vi "Lab4 prelab.vi"() -> ()   [LabVIEW 2016]
uses:
  <vilib>/Analysis/1siggen.llb/Ramp Pattern by Samples.vi
  <vilib>/Analysis/NI_AALBase.lvlib
panel:
  out "V":dbl
  out "I":dbl
  out "Data Length":dbl
  out "XY Graph":cluster{"Y":dbl[], "Y":dbl[]}[](graph)
  in  "V_D step [V]":dbl
  in  "V_D stop [V]":dbl
  in  "V_D start [V]":dbl
  in  "R":dbl
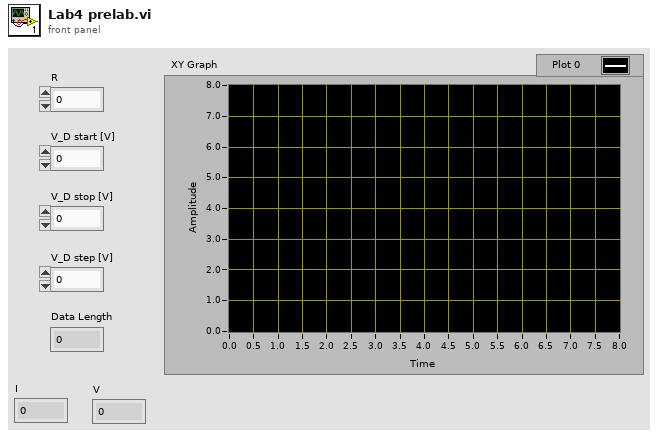
[diagram p1: front panel]
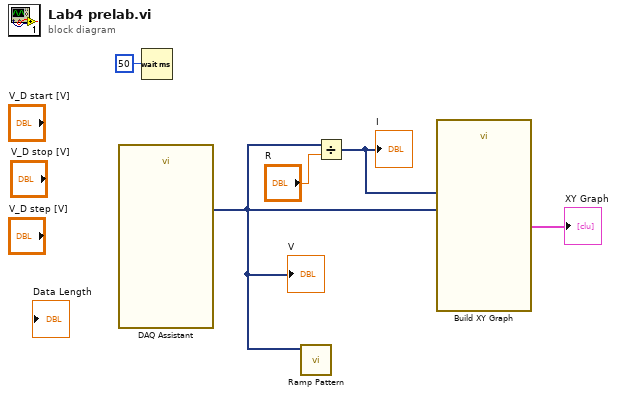
[diagram p0: block diagram]
diagram:
  n1 = call "DAQ Assistant"() -> ("data"=w1:dynamicdata)  [unwired: 17 in, 2 out]
  "V" <- w1
  n2 = Wait (ms)(milliseconds to wait=50) -> ()  [unwired: 1 out]
  n3 = call-poly <vilib>:"Ramp Pattern.vi"("samples"=w1) -> ()  [unwired: 9 in, 2 out]
  n4 = Divide(x=w1, y="R") -> (x/y=w2:dynamicdata)
  "I" <- w2
  n5 = call "Build XY Graph"("Y Input"=w1, "X Input"=w2) -> ("XY Graph"=→"XY Graph":cluster{"X":dbl[], "Y":dbl[]}[])  [unwired: 8 in, 1 out]
